vi "Self correcting directional.vi"() -> ()   [LabVIEW 2018]
uses:
  <vilib>/Studica/Studica Toolkit/Background/I2C Channel.ctl
  <vilib>/Studica/Studica Toolkit/NavX/NavX.lvlib
  CALIBRATION states.ctl
  Underlying VI's/Elasped Timer/Control.ctl
panel:
  out "Numeric":dbl
  out "State":T1
  in  "Start":bool
  out "Yaw":dbl
  in  "stop":bool
  out "Output\nSpeed":T2
  out "Output Distance":T3
  in  "xTargetSpeed":dbl
  in  "yTargetSpeed":dbl
  in  "wTargetSpeed":dbl
  in  "Zero Yaw":bool
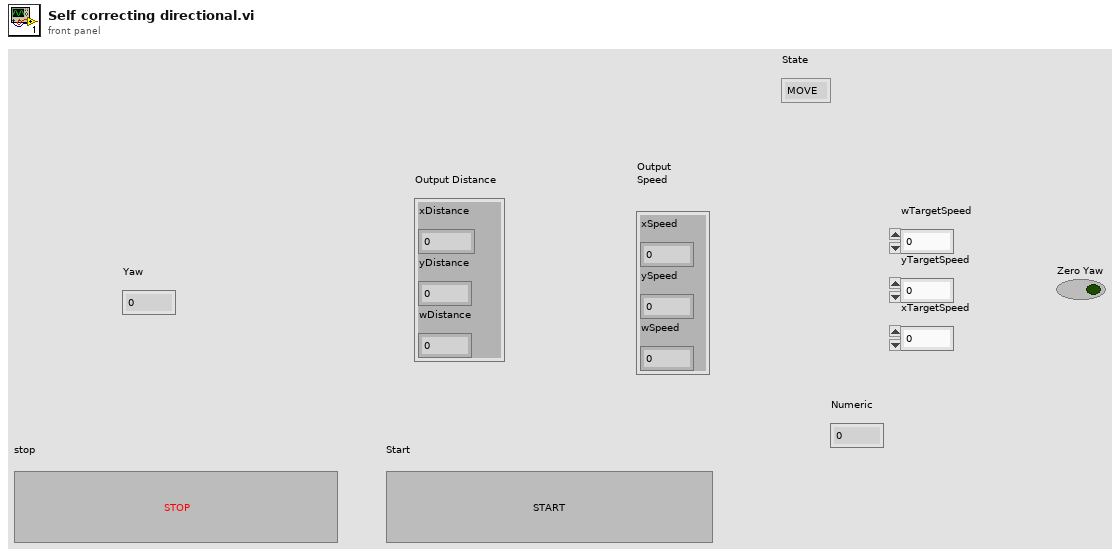
[diagram p1: front panel]
types:
  T1 = typedef "CALIBRATION states.ctl" = enum16{"MOVE", "ACW CALIBRATE", "CW CALIBRATE", "DIR CHECK", "IDLE", "INIT"}
  T2 = cluster{"xSpeed":dbl, "ySpeed":dbl, "wSpeed":dbl}
  T3 = cluster{"xDistance":dbl, "yDistance":dbl, "wDistance":dbl}
  T4 = typedef "I2C Channel.ctl" = enum16{"Not Connected", "A", "B"}
  T5 = typedef "Control.ctl" = enum16{"Start", "Pause", "Initialize"}
  T6 = cluster{"I2C Ref Out":cluster{"I2C Channel":T4, "FPGA VI Reference Out":refnum<k20>}, "Connected":bool, "Slave Address (7-bit)":u8, "Registry":u8[]}
  T7 = cluster{"Yaw":dbl, "Roll":dbl, "Pitch":dbl, "Heading":dbl, "Fused Heading":dbl}
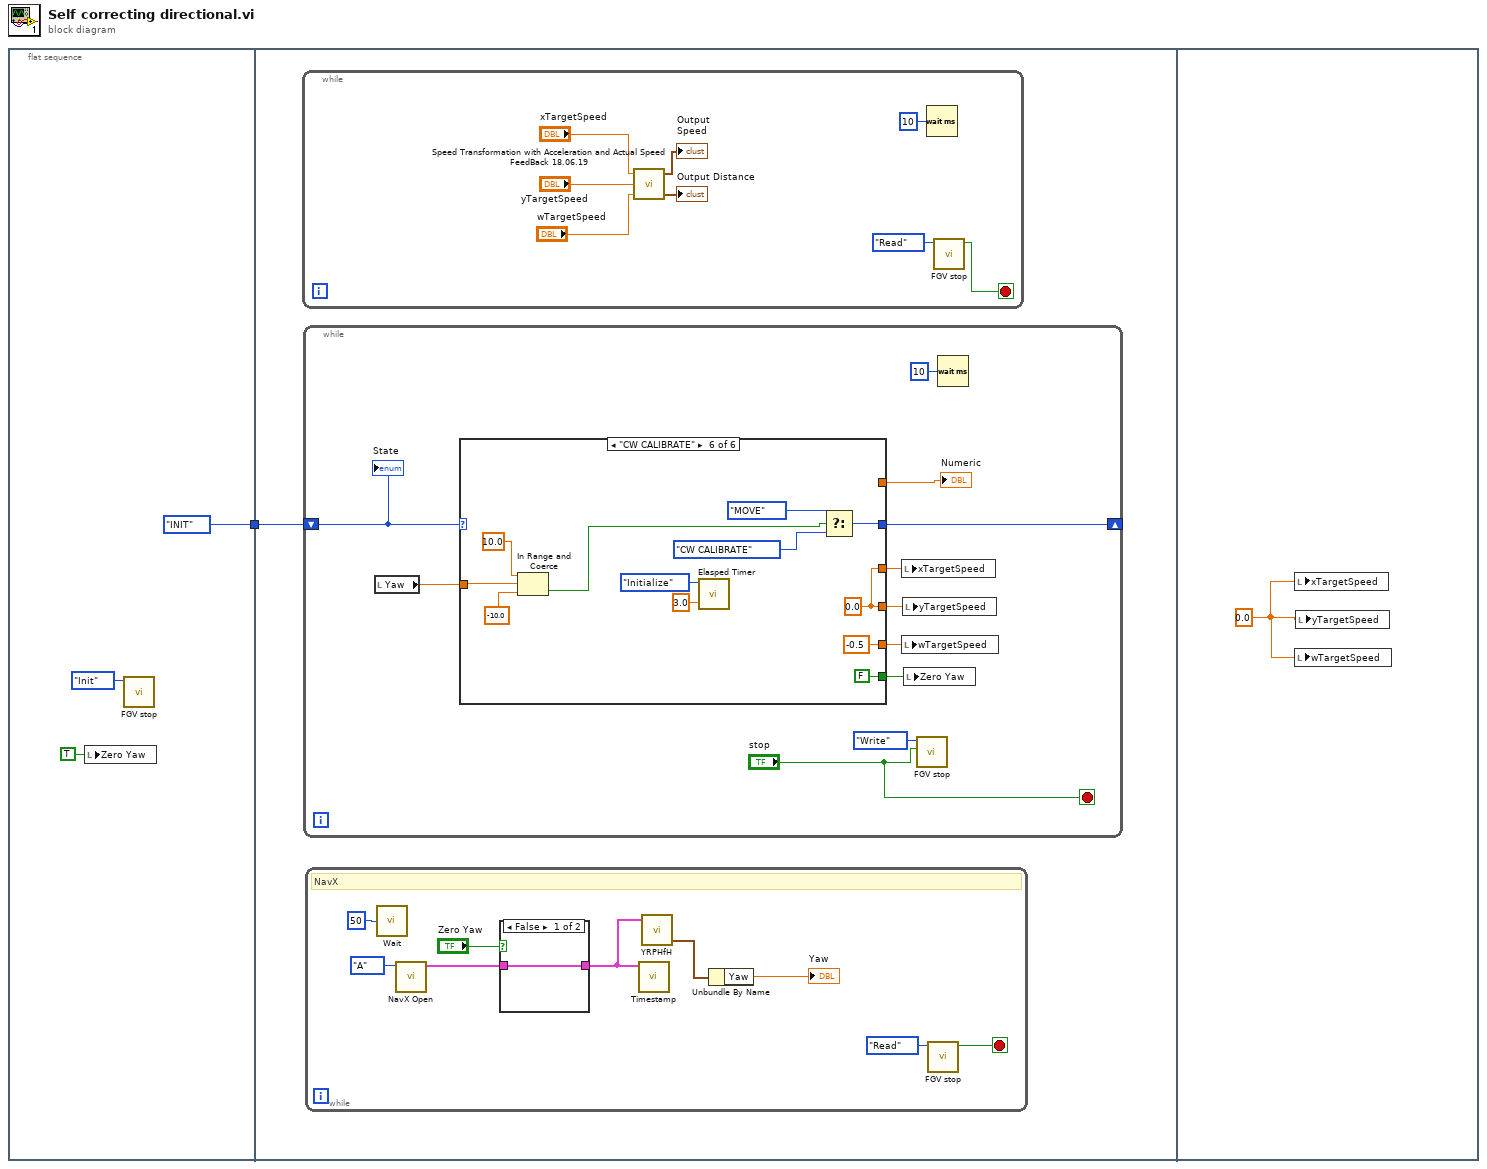
[diagram p0: block diagram]
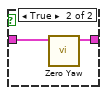
[diagram p2: hidden frame]
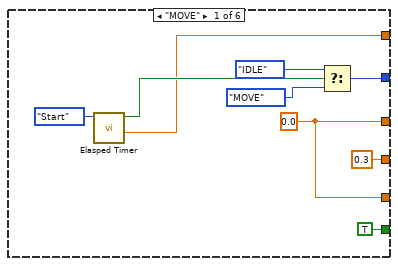
[diagram p3: hidden frame]
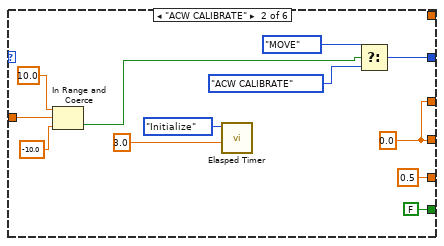
[diagram p4: hidden frame]
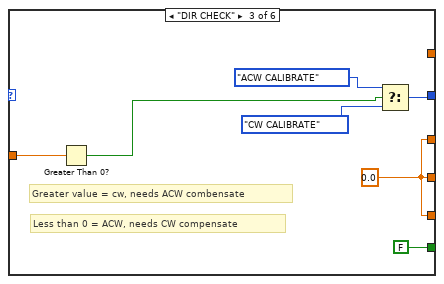
[diagram p5: hidden frame]
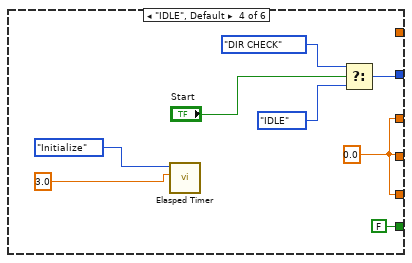
[diagram p6: hidden frame]
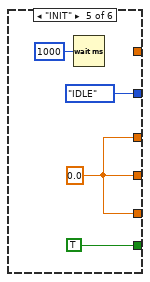
[diagram p7: hidden frame]
diagram:
  n1 = flat-sequence {
    tunnel: [CALIBRATION_states."INIT"] -> w1
    tunnel: w1 -> [w5]
    frame #0 {
      n2 = local write "Zero Yaw"(TRUE ("Zero Yaw")) -> ()
      n3 = call "FGV stop.vi"("States"=enum16{"Read", "Write", "Init"}."Init") -> ()  [unwired: 9 in, 2 out]
    }
    frame #1 {
      n4 = while {
        stop <- w13 stop-if-true
        n5 = call "Speed Transformation with Acceleration and Actual Speed FeedBack 18.06.19.vi"("wTargetSpeed"="wTargetSpeed", "yTargetSpeed"="yTargetSpeed", "xTargetSpeed"="xTargetSpeed") -> ("Output Distance"=→"Output Distance":T3, "Output\nSpeed"=→"Output\nSpeed":T2)  [unwired: 1 in]
        n6 = Wait (ms)(milliseconds to wait=u32 10) -> ()  [unwired: 1 out]
        n7 = call "FGV stop.vi"("States"=enum16{"Read", "Write", "Init"}."Read") -> ("stop Output"=w13:bool)  [unwired: 9 in, 1 out]
      }
      n8 = while {
        shift-right: [w27] -> _
        shift-left: w5 -> [w33]
        stop <- "stop" stop-if-true
        n9 = local read "Yaw"() -> (w32:dbl)
        n10 = case shown="\"CW CALIBRATE\"" w33 {
          tunnel: w32 -> [_ w54 w61 _ _ w80]
          tunnel: [0.3 w48 w59 w68 w76 w79] -> w31
          tunnel: [w39 w48 w59 w68 w76 w79] -> w30
          tunnel: [w39 0.5 w59 w68 w76 -0.5] -> w29
          tunnel: [TRUE FALSE FALSE FALSE TRUE FALSE] -> w28
          tunnel: [w45 w57 w64 w72 CALIBRATION_states."IDLE" w81] -> w27
          tunnel: [w37 _ _ _ _ _] -> w26
          frame "MOVE" {
            w39 = 0.0
            n11 = call "Elasped Timer.vi"("Action"=Control."Start") -> ("Elapsed Time"=w37:dbl, "Time Out?!"=w41:bool)  [unwired: 7 in, 2 out]
            n12 = Select(t=CALIBRATION_states."IDLE", s=w41, f=CALIBRATION_states."MOVE") -> (s? t:f=w45:T1)
          }
          frame "ACW CALIBRATE" {
            w48 = 0.0
            n13 = In Range and Coerce(upper limit=10.0, x=w54, lower limit=-10.0) -> (In Range?=w51:bool)  [unwired: 1 out]
            n14 = call "Elasped Timer.vi"("Time Setting"=3.0, "Action"=Control."Initialize") -> ()  [unwired: 6 in, 4 out]
            n15 = Select(t=CALIBRATION_states."MOVE", s=w51, f=CALIBRATION_states."ACW CALIBRATE") -> (s? t:f=w57:T1)
          }
          frame "DIR CHECK" {
            w59 = 0.0
            # "Less than 0 = ACW, needs CW compensate"
            # "Greater value = cw, needs ACW combensate"
            n16 = Greater Than 0?(x=w61) -> (x > 0?=w60:bool)
            n17 = Select(t=CALIBRATION_states."ACW CALIBRATE", s=w60, f=CALIBRATION_states."CW CALIBRATE") -> (s? t:f=w64:T1)
          }
          frame "IDLE", Default {
            w68 = 0.0
            n18 = call "Elasped Timer.vi"("Time Setting"=3.0, "Action"=Control."Initialize") -> ()  [unwired: 6 in, 4 out]
            n19 = Select(t=CALIBRATION_states."DIR CHECK", s="Start", f=CALIBRATION_states."IDLE") -> (s? t:f=w72:T1)
          }
          frame "INIT" {
            w76 = 0.0
            n20 = Wait (ms)(milliseconds to wait=u32 1000) -> ()  [unwired: 1 out]
          }
          frame "CW CALIBRATE" {
            w79 = 0.0
            n21 = In Range and Coerce(upper limit=10.0, x=w80, lower limit=-10.0) -> (In Range?=w86:bool)  [unwired: 1 out]
            n22 = call "Elasped Timer.vi"("Time Setting"=3.0, "Action"=Control."Initialize") -> ()  [unwired: 6 in, 4 out]
            n23 = Select(t=CALIBRATION_states."MOVE", s=w86, f=CALIBRATION_states."CW CALIBRATE") -> (s? t:f=w81:T1)
          }
        }
        "Numeric" <- w26
        n24 = local write "xTargetSpeed"(w30) -> ()
        n25 = local write "wTargetSpeed"(w29) -> ()
        n26 = local write "yTargetSpeed"(w31) -> ()
        n27 = local write "Zero Yaw"(w28) -> ()
        n28 = call "FGV stop.vi"("Stop Input"="stop", "States"=enum16{"Read", "Write", "Init"}."Write") -> ()  [unwired: 8 in, 2 out]
        n29 = Wait (ms)(milliseconds to wait=u32 10) -> ()  [unwired: 1 out]
        "State" <- w33
      }
      n30 = while {
        stop <- w17 stop-if-true
        # "NavX"
        n31 = call "Wait"("Count(mSec)"=u32 50) -> ()  [unwired: 1 out]
        n32 = call <vilib>:"NavX Open.vi"("I2C Channel"=I2C_Channel."A") -> ("NavX Info"=w21:T6)  [unwired: 9 in, 1 out]
        n33 = case shown="False" "Zero Yaw" {
          tunnel: w21 -> [w23 w25]
          tunnel: [w23 w24] -> w22
          frame False {
          }
          frame True {
            n34 = call <vilib>:"Zero Yaw.vi"("NavX Info In"=w25) -> ("NavX Info Out"=w24:T6)  [unwired: 10 in]
          }
        }
        n35 = call <vilib>:"Timestamp.vi"("NavX Info In"=w22) -> ()  [unwired: 9 in, 2 out]
        n36 = call <vilib>:"YRPHfH.vi"("NavX Info In"=w22) -> ("YRPHfH"=w15:T7)  [unwired: 3 in, 1 out]
        n37 = Unbundle By Name(w15) -> ("Yaw"=→"Yaw":dbl)
        n38 = call "FGV stop.vi"("States"=enum16{"Read", "Write", "Init"}."Read") -> ("stop Output"=w17:bool)  [unwired: 9 in, 1 out]
      }
    }
    frame #2 {
      w89 = 0.0
      n39 = local write "xTargetSpeed"(w89) -> ()
      n40 = local write "wTargetSpeed"(w89) -> ()
      n41 = local write "yTargetSpeed"(w89) -> ()
    }
  }
